vi "Factorysettings Pfad.vi"(8 "error in (no error)":errorcluster caption="Fehler (Eingang, kein Fehler)", 9 "Dateiname":string="abc", 11 "Ordner des Haupt-VIs":path) -> (0 "error out":errorcluster caption="Fehler (Ausgang)", 3 "Pfad Factorysettings":path)   [LabVIEW 2020, in "allgemeine Sub-VIs.lvlib"]
uses:
  allgemeine Sub-VIs.lvlib
  cRIO/SysLog/SysLog Interface cRIO.ctl
  cRIO/SysLog/SysLog_cRIO.lvlib
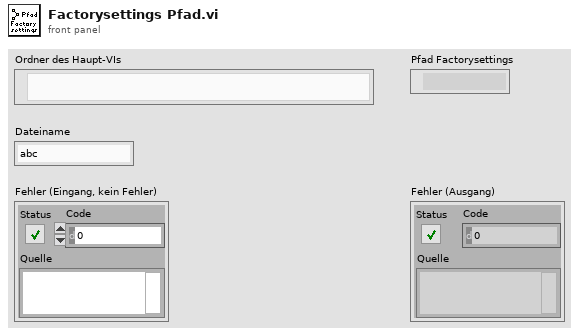
[diagram p1: front panel]
types:
  T1 = typedef "SysLog_cRIO.lvlib/SysLog Interface cRIO.ctl" = cluster{"FehlermeldungsCode":i32, "ErfolgsmeldungsCode":i32, "ParameterListenString":string, "intern":bool}
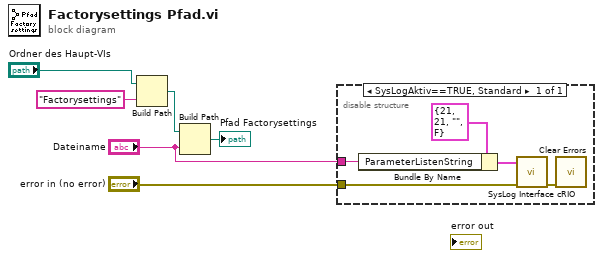
[diagram p0: block diagram]
diagram:
  n1 = Build Path(base path="Ordner des Haupt-VIs", name or relative path="Factorysettings" ("Name oder relativer Pfad")) -> (appended path=w6:path)
  n2 = Build Path(base path=w6, name or relative path="Dateiname") -> (appended path=→"Pfad Factorysettings":path)
  n3 = disable-structure shown="SysLogAktiv==TRUE, Standard" {
    disable-tunnel: "Dateiname" -> [w9]
    disable-tunnel: "error in (no error)" -> [w8]
    frame condition #0 (active) {
      n4 = Bundle By Name(cluster=T1 {"FehlermeldungsCode"=21, "ErfolgsmeldungsCode"=21, "ParameterListenString"="", "intern"=FALSE} ("Cluster (in)"), "ParameterListenString"=w9) -> (w11:T1)
      n5 = call "SysLog Interface cRIO.vi"("Fehler (in)"=w8, "Cluster (in)"=w11) -> ("Fehler (Ausgang)"=w7:errorcluster)  [unwired: 9 in]
      n6 = call <vilib>:"Clear Errors.vi"("error in (no error)"=w7) -> ()  [unwired: 5 in, 2 out]
    }
  }
